vi "Read Name.vi"(8 "error in (no error)":errorcluster, 11 "Base Step in":refnum<class "Base Step.lvclass">) -> (0 "error out":errorcluster, 2 "Name":string, 3 "Base Step out":refnum<class "Base Step.lvclass">)   [LabVIEW 2024, in "Ramses Sequencer.lvlib" / "Base Step.lvclass"]
uses:
  Base Step.lvclass
  Base Step.lvclass/Base Step.ctl
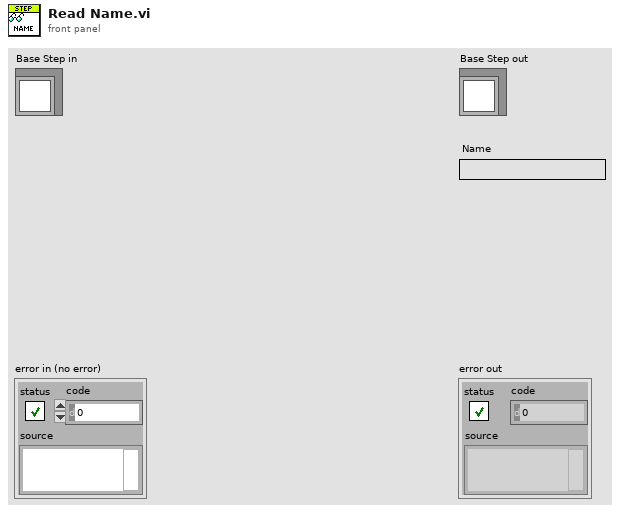
[diagram p1: front panel]
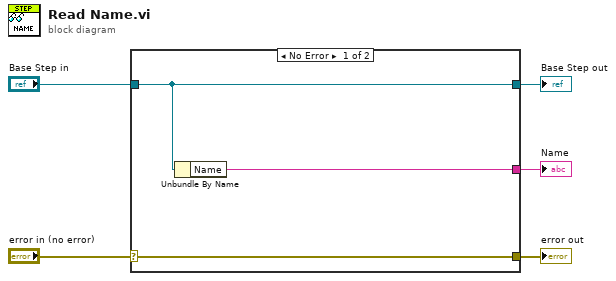
[diagram p0: block diagram]
diagram:
  n1 = case shown="No Error" "error in (no error)" {
    selector: "error in (no error)" -> [w8 w9]
    tunnel: [w8 w9] -> w4
    tunnel: [w7 w10] -> w2
    tunnel: "Base Step in" -> [w7 w10]
    tunnel: [w6 _] -> w1
    frame No Error {
      n2 = Unbundle By Name(w7) -> ("Name"=w6:string)
    }
    frame Error {
    }
  }
  "error out" <- w4
  "Base Step out" <- w2
  "Name" <- w1
